vi "HeartRate.vi"() -> ()   [LabVIEW 2020]
panel:
  out "BP (mmHg)":dbl(knob) scale=0.0..100.0
  out "Heart Rate":dbl(knob) scale=0.0..100.0
  in  "VISA resource name":refnum<visa-resource-name>
  out "Heart Rate":dbl(graph)
  out "Blood Pressure":dbl(graph)
  in  "Patient Data":string[][](table)
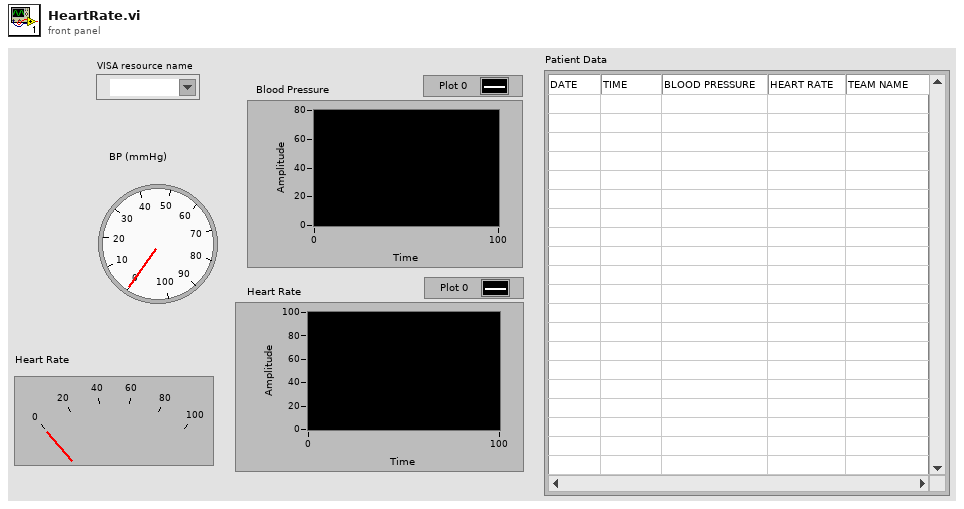
[diagram p1: front panel]
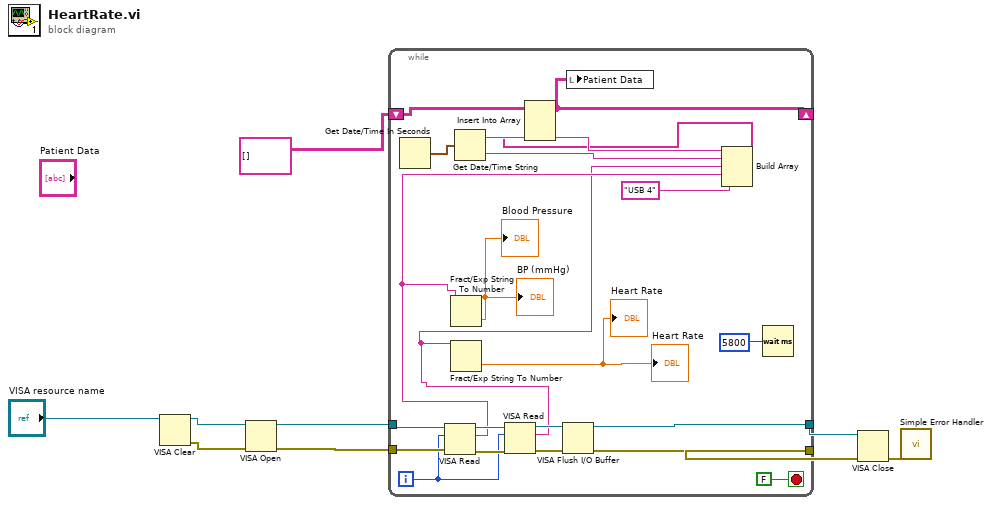
[diagram p0: block diagram]
diagram:
  n1 = VISA Clear(VISA resource name="VISA resource name") -> (VISA resource name out=w8:refnum<visa-resource-name>, error out=w7:errorcluster)  [unwired: 1 in]
  n2 = VISA Open(error in (no error)=w7, VISA resource name=w8) -> (VISA resource name=w6:refnum<visa-resource-name>, error out=w5:errorcluster)  [unwired: 3 in]
  n3 = while {
    tunnel: w6 -> [w31]
    tunnel: w5 -> [w30]
    tunnel: [w25] -> w4
    tunnel: [w24] -> w3
    shift-right: [w21] -> _
    shift-left: string[][] [] -> [w22]
    i -> [w23]
    stop <- FALSE stop-if-true
    n4 = Get Date/Time In Seconds() -> (seconds since 1Jan1904=w19:timestamp)
    n5 = VISA Read(VISA resource name=w31, byte count=w23, error in (no error)=w30) -> (VISA resource name out=w29:refnum<visa-resource-name>, read buffer=w14:string, error out=w28:errorcluster)  [unwired: 1 out]
    n6 = Fract/Exp String To Number(string=w14) -> (number=→"Blood Pressure" →"BP (mmHg)":dbl)  [unwired: 3 in, 1 out]
    n7 = Get Date/Time String(seconds (now)=w19) -> (date string=w18:string, time string=w17:string)  [unwired: 2 in]
    n8 = VISA Read(VISA resource name=w29, byte count=w23, error in (no error)=w28) -> (VISA resource name out=w27:refnum<visa-resource-name>, read buffer=w13:string, error out=w26:errorcluster)  [unwired: 1 out]
    n9 = Fract/Exp String To Number(string=w13) -> (number=→"Heart Rate" →"Heart Rate":dbl)  [unwired: 3 in, 1 out]
    n10 = VISA Flush I/O Buffer(VISA resource name=w27, error in (no error)=w26) -> (VISA resource name out=w25:refnum<visa-resource-name>, error out=w24:errorcluster)  [unwired: 1 in]
    n11 = Build Array(w18, w17, w13, w14, "USB 4" ("element")) -> (w16:string[])
    n12 = Insert Into Array(array=w22, new element=w16) -> (w21:string[][])  [unwired: 2 in]
    n13 = local write "Patient Data"(w21) -> ()
    n14 = Wait (ms)(milliseconds to wait=u32 5800) -> ()  [unwired: 1 out]
  }
  n15 = VISA Close(VISA resource name=w4, error in (no error)=w3) -> (error out=w9:errorcluster)
  n16 = call <vilib>:"Simple Error Handler.vi"("error in (no error)"=w9) -> ()  [unwired: 4 in, 5 out]
